vi "SimpleRobot_Dynamics_RevA.vi"(0 "x0":dbl, 5 "x1":dbl, 7 "y0":dbl, 9 "y1":dbl, 11 "Velocity":dbl, 12 "Direction":dbl, 13 "DeltaT (timestep)":dbl) -> (4 "x 2":dbl, 6 "y 2":dbl, 10 "Direction 2":dbl)   [LabVIEW 2010]
doc: "This subVI produces simple simulated robot dynamics"
panel:
  out "atan2(y,x)":dbl
  # "This VI calculates the Robot dynamics from frame to frame (one frame equals one time step)"
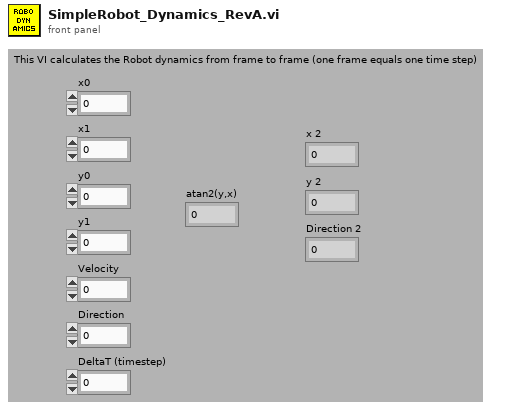
[diagram p1: front panel]
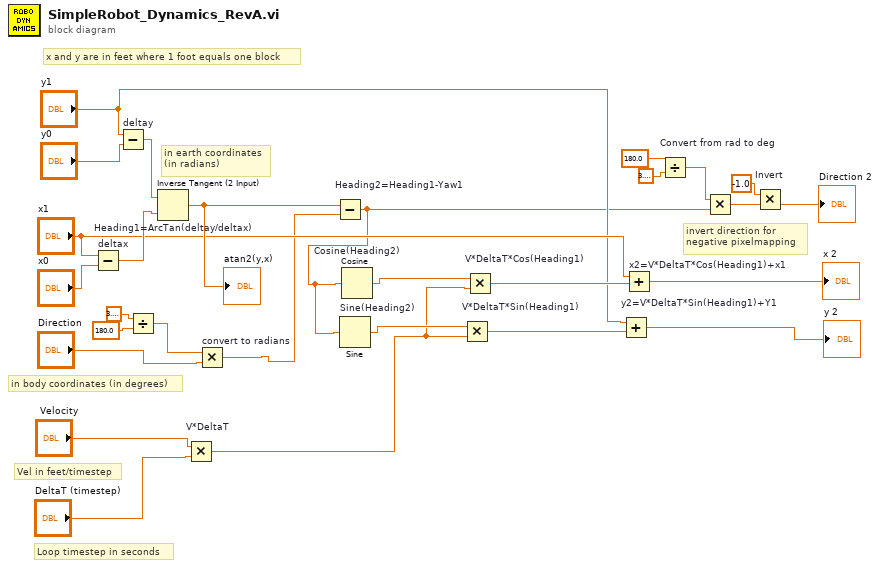
[diagram p0: block diagram]
diagram:
  # "invert direction for \nnegative pixelmapping"
  # "Loop timestep in seconds"
  # "x and y are in feet where 1 foot equals one block"
  # "Vel in feet/timestep"
  # "in earth coordinates\n(in radians)"
  # "in body coordinates (in degrees)"
  n1 = Subtract "deltax"(x="x1", y="x0") -> (x-y=w25:dbl)
  n2 = Subtract "deltay"(x="y1", y="y0") -> (x-y=w26:dbl)
  n3 = Divide(x=3.141592653589793, y=180.0) -> (x/y=w11:dbl)
  n4 = Inverse Tangent (2 Input) "Heading1=ArcTan(deltay/deltax)"(1:w25, 2:w26) -> (0:w24:dbl)
  "atan2(y,x)" <- w24
  n5 = Multiply "V*DeltaT"(x="Velocity", y="DeltaT (timestep)") -> (x*y=w20:dbl)
  n6 = Multiply "convert to radians"(x=w11, y="Direction") -> (x*y=w1:dbl)
  n7 = Subtract "Heading2=Heading1-Yaw1"(x=w24, y=w1) -> (x-y=w5:dbl)
  n8 = Sine "Sine(Heading2)"(x=w5) -> (sin(x)=w21:dbl)
  n9 = Cosine "Cosine(Heading2)"(x=w5) -> (cos(x)=w22:dbl)
  n10 = Multiply "V*DeltaT*Sin(Heading1)"(x=w21, y=w20) -> (x*y=w16:dbl)
  n11 = Multiply "V*DeltaT*Cos(Heading1)"(x=w22, y=w20) -> (x*y=w19:dbl)
  n12 = Add "y2=V*DeltaT*Sin(Heading1)+Y1"(x="y1", y=w16) -> (x+y=→"y 2":dbl)
  n13 = Add "x2=V*DeltaT*Cos(Heading1)+x1"(x="x1", y=w19) -> (x+y=→"x 2":dbl)
  n14 = Divide "Convert from rad to deg"(x=180.0, y=3.141592653589793) -> (x/y=w7:dbl)
  n15 = Multiply(x=w7, y=w5) -> (x*y=w2:dbl)
  n16 = Multiply "Invert"(x=-1.0, y=w2) -> (x*y=→"Direction 2":dbl)
